vi "PC_Test_Network_Streams.vi"() -> ()   [LabVIEW 2020]
uses:
  <vilib>/dex/Stream Element Allocation Mode.ctl
  <vilib>/Waveform/WDTOps.llb/WDT Get Final Time Value DBL.vi
panel:
  in  "stop":bool
  out "Waveform Chart 2":waveform(dbl)(graph)
  out "Waveform Chart":waveform(i32)(graph)
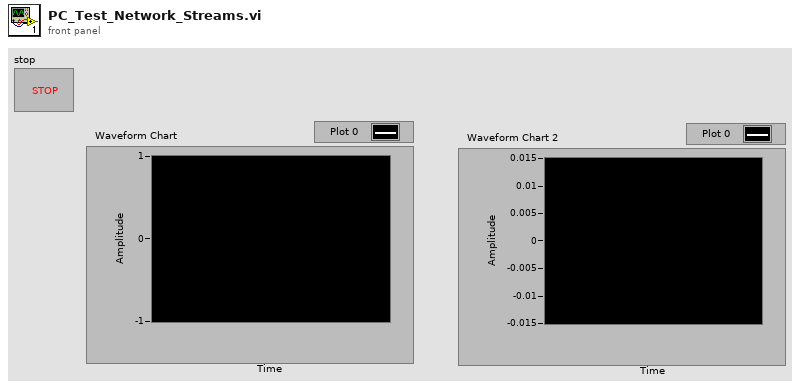
[diagram p1: front panel]
types:
  T1 = typedef "Stream Element Allocation Mode.ctl" = u32
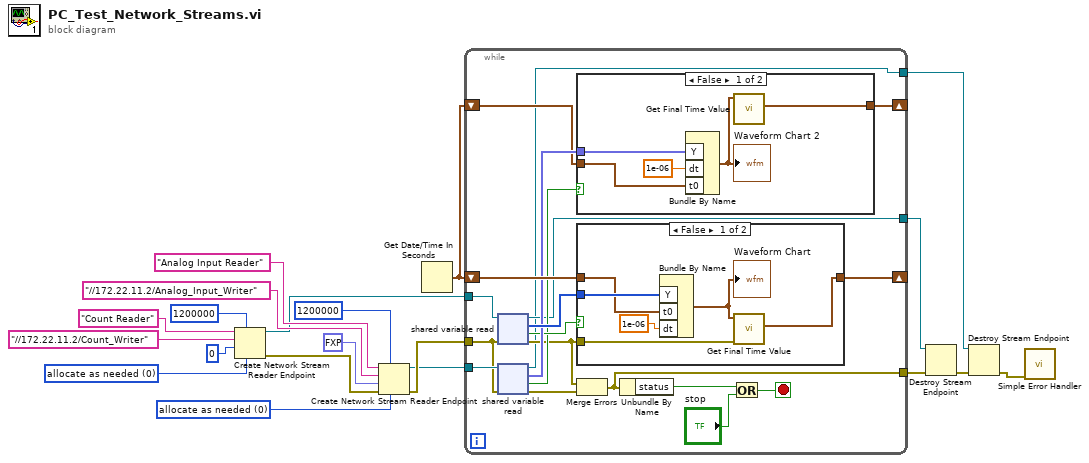
[diagram p0: block diagram]
diagram:
  w14 = T1 0 items=["allocate as needed", "pre-allocate"] ("element allocation mode")
  w17 = T1 0 items=["allocate as needed", "pre-allocate"] ("element allocation mode")
  n1 = Create Network Stream Reader Endpoint(6:w17, 7:1200000 ("reader buffer size"), 9:0, 10:"//172.22.11.2/Count_Writer" ("writer url"), 11:"Count Reader" ("reader name")) -> (0:w11:errorcluster, 3:w10:refnum<k21>)  [unwired: 2 in]
  n2 = Create Network Stream Reader Endpoint(6:w14, 7:1200000 ("reader buffer size"), 8:w11, 9:fxp<+/-,17,5> 0.0, 10:"//172.22.11.2/Analog_Input_Writer" ("writer url"), 11:"Analog Input Reader" ("reader name")) -> (0:w9:errorcluster, 3:w8:refnum<k21>)  [unwired: 1 in]
  n3 = Get Date/Time In Seconds() -> (seconds since 1Jan1904=w6:timestamp)
  n4 = while {
    shift-right: [w36] -> _
    shift-left: w6 -> [w37]
    tunnel: w10 -> [w39]
    tunnel: w9 -> [w34]
    tunnel: w8 -> [w35]
    shift-right: [w31] -> _
    shift-left: w6 -> [w32]
    tunnel: [w23] -> w4
    tunnel: [w22] -> w5
    tunnel: [w21] -> w3
    stop <- w24 stop-if-true
    n5 = shared-variable-read(w39, w34) -> (w22:refnum<k21>, w28:errorcluster, w30:bool, w38:i32[])  [unwired: 2 in]
    n6 = shared-variable-read(w35, w34) -> (w21:refnum<k21>, w27:errorcluster, w29:bool, w33:fxp<+/-,17,5>[])  [unwired: 2 in]
    n7 = case shown="False" w29 {
      tunnel: w33 -> [w44 _]
      tunnel: w32 -> [w42 w45]
      tunnel: [w41 w45] -> w31
      frame False {
        n8 = Bundle By Name("Y"=w44, "dt"=1e-06, "t0"=w42) -> (w40:waveform(dbl))  [unwired: 1 in]
        "Waveform Chart 2" <- w40
        n9 = call-poly <vilib>:"Get Final Time Value.vi"("waveform in"=w40) -> ("tf"=w41:timestamp)  [unwired: 8 in, 2 out]
      }
      frame True {
      }
    }
    n10 = case shown="False" w30 {
      tunnel: w38 -> [w51 _]
      tunnel: w37 -> [w50 w52]
      tunnel: [w47 w52] -> w36
      tunnel: w28 -> [w46 _]
      frame False {
        n11 = Bundle By Name("Y"=w51, "t0"=w50, "dt"=1e-06) -> (w48:waveform(i32))  [unwired: 1 in]
        "Waveform Chart" <- w48
        n12 = call-poly <vilib>:"Get Final Time Value.vi"("error in (no error)"=w46, "waveform in"=w48) -> ("tf"=w47:timestamp)  [unwired: 7 in, 2 out]
      }
      frame True {
      }
    }
    n13 = Merge Errors(w28, w27) -> (w23:errorcluster)
    n14 = Unbundle By Name(w23) -> ("status"=w25:bool)
    n15 = Or(x=w25, y="stop") -> (x .or. y?=w24:bool)
  }
  n16 = Destroy Stream Endpoint(8:w4, 11:w5) -> (0:w2:errorcluster)
  n17 = Destroy Stream Endpoint(8:w2, 11:w3) -> (0:w1:errorcluster)
  n18 = call <vilib>:"Simple Error Handler.vi"("error in (no error)"=w1) -> ()  [unwired: 4 in, 5 out]
